vi "PIL_Main.vi"() -> ()   [LabVIEW 2018]
uses:
  controls/EXPERIMENT_Inputs.ctl
  controls/LASER_Inputs.ctl
  controls/LAMP_Inputs.ctl
  controls/GAS_Inputs.ctl
  controls/EXPERT_Inputs.ctl
  controls/DIGIT_5122_Inputs.ctl
  <instrlib>/niScope/Controls/niScope trigger source.ctl
  controls/HSDIO_6541_Inputs.ctl
  <instrlib>/niHSDIO/niHSDIO.llb/niHSDIO_ctl Trigger Source Values (Ring).ctl
  controls/SOFTWARE_Inputs.ctl
  controls/AO_6711_Inputs.ctl
  controls/AWG_5421_Inputs.ctl
  <instrlib>/niFgen/niFgen.llb/niFgen_ctl Trigger Source Values (Ring).ctl
  controls/XML_Inputs.ctl
  controls/VOLTAGES_Inputs.ctl
  controls/HEXA_Inputs.ctl
  controls/QUAD_Inputs.ctl
  controls/SEQUENCE_Inputs.ctl
  controls/EXCIT_Inputs.ctl
  controls/DATA_Inputs.ctl
  controls/TIMING_Inputs.ctl
  controls/PROCESSING_Inputs.ctl
  controls/TRAPPING_Inputs.ctl
  controls/SPECTRUM.ctl
  controls/EXCIT_Table.ctl
  controls/TIMING_Table.ctl
  controls/TIMING_Mandatory_Items.ctl
  controls/TIMING_Optional_Items.ctl
  controls/PIL_Status.ctl
  controls/QMH_UI_Cluster.ctl
  controls/QMH_UI_References.ctl
  controls/QMH_UI_Report.ctl
  controls/QMH_UI_Command.ctl
  controls/QMH_ICR_Command.ctl
  controls/QMH_Status.ctl
  controls/EXPERT_Path_Selector.ctl
  <vilib>/Utility/error.llb/DialogType.ctl
  Global_Variables.vi
panel:
  in  "Save As":bool
  in  "error in (no error)":errorcluster
  in  "Start":bool
  in  "Load":bool
  in  "Exit":bool
  in  "Tabs":T1(tab)
  out "SPECTRUM":T2={"Day Path"=path "D:/PIRENEA/DATA/2016/data_2016_01_01", "Spectrum Name"="2016_01_01_000.A00", "Accumulated"=FALSE, "Stored in Database"=FALSE, "From a Set of"=0, "Quality Flag"="Optimal"}
  in  "Change Experiment":bool
  out "EXPERIMENT Inputs":T3={"Setup"="", "Date"="", "User Name"="", "Comment"="", "Experiment Procedures"=[], "Chemical Source"="", "Sample Components"=[], "Species"=[], "Laser 1"={"Used"=TRUE, "Name"="Spectroscopy", "Wavelength"=1000.0, "Energy"=25.0}, "Laser 2"={"Used"=TRUE, "Name"="Spectroscopy", "Wavelength"=1000.0, "Energy"=25.0}, "Laser 3"={"Used"=TRUE, "Name"="Spectroscopy", "Wavelength"=1000.0, "Energy"=25.0}, "Laser 4"={"Used"=TRUE, "Name"="Spectroscopy", "Wavelength"=1000.0, "Energy"=25.0}, "Laser 5"={"Used"=TRUE, "Name"="Spectroscopy", "Wavelength"=1000.0, "Energy"=25.0}, "Lamp 1"={"Used"=TRUE, "Name"="Spectroscopy", "Wavelength"=1000.0, "Attenuation"=25.0}, "Lamp 2"={"Used"=TRUE, "Name"="Spectroscopy", "Wavelength"=1000.0, "Attenuation"=25.0}, "Gas 1"={"Used"=TRUE, "Name"="Spectroscopy", "Pressure"=1000.0}, "Gas 2"={"Used"=TRUE, "Name"="Spectroscopy", "Pressure"=1000.0}, "Gas 3"={"Used"=TRUE, "Name"="Spectroscopy", "Pressure"=1000.0}, "Gas 4"={"Used"=TRUE, "Name"="Spectroscopy", "Pressure"=1000.0}, "Gas 5"={"Used"=TRUE, "Name"="Spectroscopy", "Pressure"=1000.0}} caption="EXCIT Paths"
  in  "Change Voltages":bool
  out "VOLTAGES Inputs":T7={"Hexa 1"={"Used"=FALSE, "Voltage"=0.0}, "Hexa 2"={"Used"=FALSE, "Voltage"=0.0}, "Hexa 3"={"Used"=FALSE, "Voltage"=0.0}, "Quad 1"={"Used"=TRUE, "Voltage"=25.0}, "Quad 2"={"Used"=TRUE, "Voltage"=25.0}, "Quad 3"={"Used"=TRUE, "Voltage"=25.0}}
  out "SEQUENCE Inputs":T10={"EXCIT Inputs"={"Number of Excitations"=1, "Script Text"="script  excit1wfm\r    wait until scriptTrigger0\r    generate Sinus250to500a25dur1200fs10\rend script", "Table of Waveforms"=["Sinus250to500a25dur1200fs10"]}, "DATA Inputs"={"Record Length"=524000, "Sample Rate"=2000000.0, "Data Type"=0, "Vertical Range"=2.0, "Acquisition Duration"=100000.0}, "TIMING Inputs"={"Number of Acquisitions "=1, "Number of Accumulations"=1, "Table of Waveforms"=["", "", "", "", "", "", "", "", "", "", "", ""], "Script Text"=""}, "PROCESSING Inputs"={"Reference Mass"=300.0939, "Cyclotron Freq"=255.727, "Magnetron Freq"=0.001}, "TRAPPING Inputs"={"Number of Channels"=4, "Init Values"=[2.0, 9.0, 9.0, 2.0], "Opening Values"=[0.0, 0.0, 0.0, 0.0], "Trapping Values"=[2.0, 9.0, 9.0, 2.0], "Emptying Values"=[-10.0, -10.0, -10.0, -10.0], "Adiabatic ON"=FALSE, "Adiabatic Duration"=0, "Adiabatic Waveforms"=["Adiabatic_None_2_2_2000", "Adiabatic_Ramp_9_0_2000", "Adiabatic_DoubleRamp_9_0_2000", "Adiabatic_RC_2_0_2000.bin"], "Ions Refill ON"=FALSE, "Number of Ions Refills"=4, "Trapping Delay"=400.0, "Trapping Duration"=300.0}} {"TRAPPING Inputs"."Trapping Duration" min=2.0; "TRAPPING Inputs"."Trapping Delay" min=2.0; "TRAPPING Inputs"."Number of Ions Refills" min=1 max=1000; "TRAPPING Inputs"."Trapping Values" min=-10.0 max=10.0; "TRAPPING Inputs"."Init Values" min=-10.0 max=10.0; "TRAPPING Inputs"."Emptying Values" min=-10.0 max=10.0; "TRAPPING Inputs"."Opening Values" min=-10.0 max=10.0; "PROCESSING Inputs"."Magnetron Freq" format="%.5g"; "PROCESSING Inputs"."Cyclotron Freq" format="%.5g"; "PROCESSING Inputs"."Reference Mass" format="%.5g"; "TIMING Inputs"."Number of Accumulations" min=0 max=50 step=1; "TIMING Inputs"."Number of Acquisitions" min=1 max=10 step=1; "DATA Inputs"."Vertical Range" items=["0.2"=0.2, "0.4"=0.4, "1"=1.0, "2"=2.0, "4"=4.0, "10"=10.0]; "DATA Inputs"."Data Type" items=["I16", "DBL"]; "DATA Inputs"."Sample Rate" items=["1 MHz"=1000000.0, "2 MHz"=2000000.0, "5 MHz"=5000000.0, "10 MHz"=10000000.0, "20 MHz"=20000000.0, "25 MHz"=25000000.0, "50 MHz"=50000000.0, "100 MHz"=100000000.0]; "EXCIT Inputs"."Number of Excitations" min=1 max=10}
  in  "Change Sequence":bool
  in  "Change Expert":bool
  out "EXPERT Inputs":T16={"DIGIT 5122 Inputs"={"Sample Rate"=5000000.0, "Resource Name"="DIGIT_5122", "Channel Name"="0", "Trigger Source"="VAL_EXTERNAL", "Vertical Range"=2.0, "Trigger Level"=3.0}, "HSDIO 6541 Inputs"={"Resource Name"="HSDIO_6541", "Clock Rate"=1000000.0, "Trigger Source"="PFI0"}, "SOFTWARE Inputs"={"Application Directory"=path "D:/S.O.F.T.S/LABVIEW/PIL", "Software Version"="17.0f2", "Data Path"=path "D:/PIRENEA/DATA", "XML Path"=path "D:/PIRENEA/DATA", "XML File Filter"="*.xml", "XML Saved Path"=path "D:/PIRENEA/SAVED_XML", "Excit Scripts Path"=path "D:/PIRENEA/TECHNICAL/EXCIT_SCRIPTS", "Excit Scripts File Filter"="*.txt", "Excit Waveforms Path"=path "D:/PIRENEA/TECHNICAL/EXCIT_WFMS", "Excit Waveforms File Filter"="*.bin", "Timing Scripts Path"=path "D:/PIRENEA/TECHNICAL/TIMING_SCRIPTS", "Timing Scripts File Filter"="*.txt", "Timing Waveforms Path"=path "D:/PIRENEA/TECHNICAL/TIMING_WFMS", "Timing Waveforms File Filter"="*.bin", "Trapping Waveforms Path"=path "D:/PIRENEA/TECHNICAL/TRAPPING_WFMS", "Trapping Waveforms File Filter"="*.bin"}, "AO 6711 Inputs"={"Physical Channels"="AO_6711/ao0:3", "Min Voltage"=-10.0, "Max Voltage"=10.0, "Trigger Source"="/AO_6711/PFI3", "Counter"="AO_6711/ctr0"}, "AWG 5421 Inputs"={"Resource Name"="AWG_5421", "Sample Rate"=10000000.0, "Trigger Type"=2, "Trigger Source"="PFI0", "Waveform Gain"=0.31, "Digital Filter ON"=TRUE}, "XML Inputs"={"Version Tag Name"="XML_Version", "Version String"="1.1"}} {"AWG 5421 Inputs"."Sample Rate" format="%.2p"; "AWG 5421 Inputs"."Trigger Type" items=["None", "Software Edge", "Digital Edge", "Digital Level"]; "AO 6711 Inputs"."Max Voltage" min=-10.0 max=10.0; "AO 6711 Inputs"."Min Voltage" min=-10.0 max=10.0; "HSDIO 6541 Inputs"."Clock Rate" format="%.2p"; "DIGIT 5122 Inputs"."Trigger Level" format="%.2f"; "DIGIT 5122 Inputs"."Vertical Range" format="%.2f"; "DIGIT 5122 Inputs"."Sample Rate" step=65535.0 format="%#_3p"}
  in  "Excit Test":bool caption="AWG5421 Board"
  out "TIMING Script":string
  in  "Change Scientist":bool
  out "TIMING Table":T26={"Mandatory Items"={"Script Name"="", "GINI Time Period"=100.0, "HSDIO Delay"=60.0, "Shutter Duration before"=50.0, "Shutter Duration after"=50.0, "Filter Tau"=2.0, "Emtyping Duration"=1000.0}, "Optional Items"={"Eject"=0, "Acq"=0, "Excit"=0, "Gas"=0, "Laser"=0, "Lamp"=0}, "Times Table"=[["Excit1", "name", "Swift", "0.5", "1200", "70", "150", "550", "0", "0", "0"]]} {"Optional Items"."Laser" min=0 max=3; "Optional Items"."Gas" min=0 max=5; "Mandatory Items"."GINI Time Period" min=100000.0 max=1000000.0 format="%#_7g"; "Mandatory Items"."Shutter Duration after" min=2.0 max=100000.0; "Mandatory Items"."HSDIO Delay" min=0.0 max=100.0; "Mandatory Items"."Shutter Duration before" min=2.0 max=100000.0; "Mandatory Items"."Filter Tau" min=1000.0 max=2000.0; "Mandatory Items"."Emtyping Duration" min=2.0 format="%#_8g"}
  out "EXCIT Table":T29={"Number of Excits"=0, "Number of Ejects"=0, "Sampling Frequency"=0.0, "Waveforms Table"=[["Excit1", "name", "Swift", "0.5", "1200", "70", "150", "550", "0", "0", "0"]]}
  out "PIL Status":T30
  # "Lasers"
  # "nm"
  # "mJ"
  # "Lamps"
  # "nm"
  # "dB"
  # "Gas"
  # "bar"
  # "HEXAPOLE"
  # "QUADRIPOLE"
  # "GO_out"
  # "Gout"
  # "GI_in"
  # "Gin"
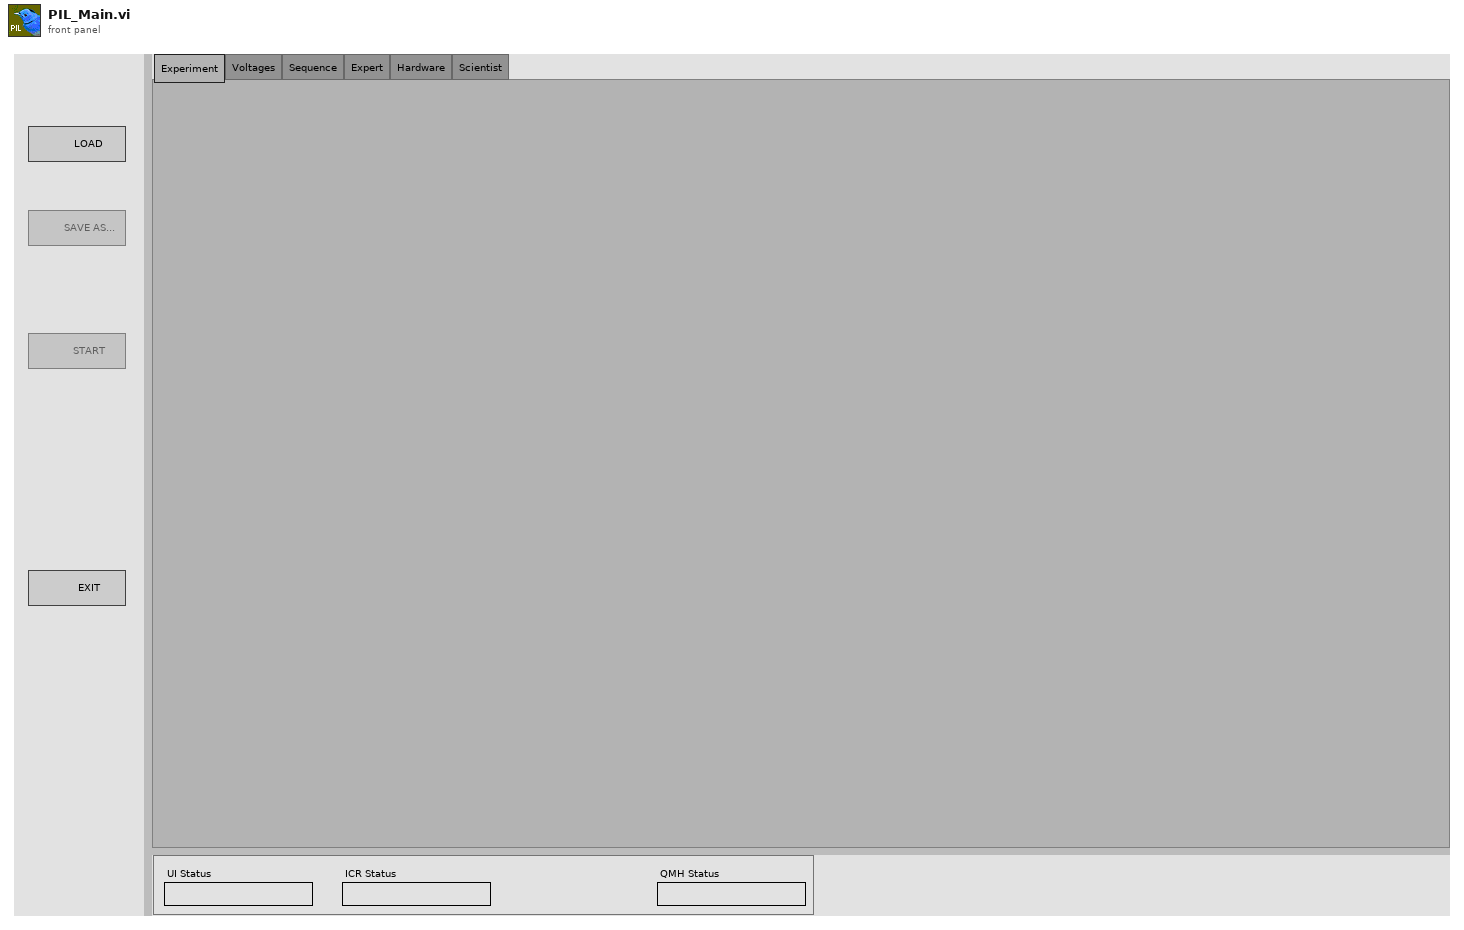
[diagram p1: front panel]
types:
  T1 = enum32{"Experiment", "Voltages", "Sequence", "Expert", "Hardware", "Scientist"}
  T2 = typedef "SPECTRUM.ctl" = cluster{"Day Path":path, "Spectrum Name":string, "Accumulated":bool, "Stored in Database":bool, "From a Set of":i16, "Quality Flag":string}
  T3 = typedef "EXPERIMENT_Inputs.ctl" = cluster{"Setup":string, "Date":string, "User Name":string, "Comment":string, "Experiment Procedures":string[], "Chemical Source":string, "Sample Components":string[], "Species":string[], "Laser 1":T4, "Laser 2":T4, "Laser 3":T4, "Laser 4":T4, "Laser 5":T4, "Lamp 1":T5, "Lamp 2":T5, "Gas 1":T6, "Gas 2":T6, "Gas 3":T6, "Gas 4":T6, "Gas 5":T6}
  T4 = typedef "LASER_Inputs.ctl" = cluster{"Used":bool, "Name":string, "Wavelength":dbl, "Energy":dbl}
  T5 = typedef "LAMP_Inputs.ctl" = cluster{"Used":bool, "Name":string, "Wavelength":dbl, "Attenuation":dbl}
  T6 = typedef "GAS_Inputs.ctl" = cluster{"Used":bool, "Name":string, "Pressure":dbl}
  T7 = typedef "VOLTAGES_Inputs.ctl" = cluster{"Hexa 1":T8, "Hexa 2":T8, "Hexa 3":T8, "Quad 1":T9, "Quad 2":T9, "Quad 3":T9}
  T8 = typedef "HEXA_Inputs.ctl" = cluster{"Used":bool, "Voltage":dbl}
  T9 = typedef "QUAD_Inputs.ctl" = cluster{"Used":bool, "Voltage":dbl}
  T10 = typedef "SEQUENCE_Inputs.ctl" = cluster{"EXCIT Inputs":T11, "DATA Inputs":T12, "TIMING Inputs":T13, "PROCESSING Inputs":T14, "TRAPPING Inputs":T15}
  T11 = typedef "EXCIT_Inputs.ctl" = cluster{"Number of Excitations":i32, "Script Text":string, "Table of Waveforms":string[]}
  T12 = typedef "DATA_Inputs.ctl" = cluster{"Record Length":i32, "Sample Rate":dbl, "Data Type":u8, "Vertical Range":dbl, "Acquisition Duration":dbl}
  T13 = typedef "TIMING_Inputs.ctl" = cluster{"Number of Acquisitions ":i16, "Number of Accumulations":i16, "Table of Waveforms":string[], "Script Text":string}
  T14 = typedef "PROCESSING_Inputs.ctl" = cluster{"Reference Mass":dbl, "Cyclotron Freq":dbl, "Magnetron Freq":dbl}
  T15 = typedef "TRAPPING_Inputs.ctl" = cluster{"Number of Channels":i32, "Init Values":dbl[], "Opening Values":dbl[], "Trapping Values":dbl[], "Emptying Values":dbl[], "Adiabatic ON":bool, "Adiabatic Duration":i32, "Adiabatic Waveforms":string[], "Ions Refill ON":bool, "Number of Ions Refills":i32, "Trapping Delay":dbl, "Trapping Duration":dbl}
  T16 = typedef "EXPERT_Inputs.ctl" = cluster{"DIGIT 5122 Inputs":T17, "HSDIO 6541 Inputs":T19, "SOFTWARE Inputs":T21, "AO 6711 Inputs":T22, "AWG 5421 Inputs":T23, "XML Inputs":T25}
  T17 = typedef "DIGIT_5122_Inputs.ctl" = cluster{"Sample Rate":dbl, "Resource Name":refnum<k15>, "Channel Name":string, "Trigger Source":T18, "Vertical Range":dbl, "Trigger Level":dbl}
  T18 = typedef "niScope trigger source.ctl" = string
  T19 = typedef "HSDIO_6541_Inputs.ctl" = cluster{"Resource Name":refnum<k15>, "Clock Rate":dbl, "Trigger Source":T20}
  T20 = typedef "niHSDIO_ctl Trigger Source Values (Ring).ctl" = string
  T21 = typedef "SOFTWARE_Inputs.ctl" = cluster{"Application Directory":path, "Software Version":string, "Data Path":path, "XML Path":path, "XML File Filter":string, "XML Saved Path":path, "Excit Scripts Path":path, "Excit Scripts File Filter":string, "Excit Waveforms Path":path, "Excit Waveforms File Filter":string, "Timing Scripts Path":path, "Timing Scripts File Filter":string, "Timing Waveforms Path":path, "Timing Waveforms File Filter":string, "Trapping Waveforms Path":path, "Trapping Waveforms File Filter":string}
  T22 = typedef "AO_6711_Inputs.ctl" = cluster{"Physical Channels":tag, "Min Voltage":dbl, "Max Voltage":dbl, "Trigger Source":tag, "Counter":tag}
  T23 = typedef "AWG_5421_Inputs.ctl" = cluster{"Resource Name":refnum<k15>, "Sample Rate":dbl, "Trigger Type":u16, "Trigger Source":T24, "Waveform Gain":dbl, "Digital Filter ON":bool}
  T24 = typedef "niFgen_ctl Trigger Source Values (Ring).ctl" = string
  T25 = typedef "XML_Inputs.ctl" = cluster{"Version Tag Name":string, "Version String":string}
  T26 = typedef "TIMING_Table.ctl" = cluster{"Mandatory Items":T27, "Optional Items":T28, "Times Table":string[][]}
  T27 = typedef "TIMING_Mandatory_Items.ctl" = cluster{"Script Name":string, "GINI Time Period":dbl, "HSDIO Delay":dbl, "Shutter Duration before":dbl, "Shutter Duration after":dbl, "Filter Tau":dbl, "Emtyping Duration":dbl}
  T28 = typedef "TIMING_Optional_Items.ctl" = cluster{"Eject":u32, "Acq":i32, "Excit":u32, "Gas":i32, "Laser":i32, "Lamp":i32}
  T29 = typedef "EXCIT_Table.ctl" = cluster{"Number of Excits":u16, "Number of Ejects":u16, "Sampling Frequency":dbl, "Waveforms Table":string[][]}
  T30 = typedef "PIL_Status.ctl" = cluster{"UI Status":string, "ICR Status":string, "QMH Status":string}
  T31 = typedef "QMH_UI_Cluster.ctl" = cluster{"QMH UI References":T32, "QMH UI Report":T33}
  T32 = typedef "QMH_UI_References.ctl" = cluster{"Refnum Load":refnum<vi>, "Refnum Save As":refnum<vi>, "Refnum Start":refnum<vi>, "Refnum Exit":refnum<vi>, "Refnum Tabs":refnum<vi>, "Refnum SPECTRUM":refnum<vi>, "Refnum EXPERIMENT":refnum<vi>, "Refnum VOLTAGES":refnum<vi>, "Refnum SEQUENCE":refnum<vi>, "Refnum EXPERT":refnum<vi>, "Refnum EXCIT Table":refnum<vi>, "Refnum TIMING Table":refnum<vi>, "Refnum CHANGE Experiment":refnum<vi>, "Refnum CHANGE Voltages":refnum<vi>, "Refnum CHANGE Sequence":refnum<vi>, "Refnum CHANGE Expert":refnum<vi>, "Refnum CHANGE Scientist":refnum<vi>, "Refnum PIL Status":refnum<vi>}
  T33 = typedef "QMH_UI_Report.ctl" = cluster{"UI Status":T34, "ICR Status":T35, "QMH Status":T36}
  T34 = typedef "QMH_UI_Command.ctl" = enum16{"Initialize", "UI Load", "UI Save", "UI Save As", "UI Change Experiment", "UI Change Voltages", "UI Change Sequence", "UI Change Expert", "UI Change Scientist", "Ready to Start", "UI Start", "Waiting for ICR", "UI Exit", "Update Report", "Update ICR Status", "Waiting for User"}
  T35 = typedef "QMH_ICR_Command.ctl" = enum16{"Initialize", "Sequence Setup", "ICR Start", "ICR Stop", "Hardware Setup", "Next Accumulation", "Waiting for Trigger", "Sequence Started", "Sequence Finished", "Writing Data", "Hardware Reset", "Exit"}
  T36 = typedef "QMH_Status.ctl" = enum16{"Init", "Loading", "Setup", "Ready to Start", "Started", "Idle"}
  T37 = typedef "EXPERT_Path_Selector.ctl" = enum16{"Application", "Resources", "Data", "XML", "XML Saved", "Load Directory"}
  T38 = typedef "QMH_UI_Message.ctl" = cluster{"Command":T34, "Data":variant}
  T39 = typedef "DialogType.ctl" = u16
  T40 = enum32{"invalid app kind", "Development System", "Run Time System", "Student Edition", "Embedded LabVIEW", "Evaluation", "Custom"}
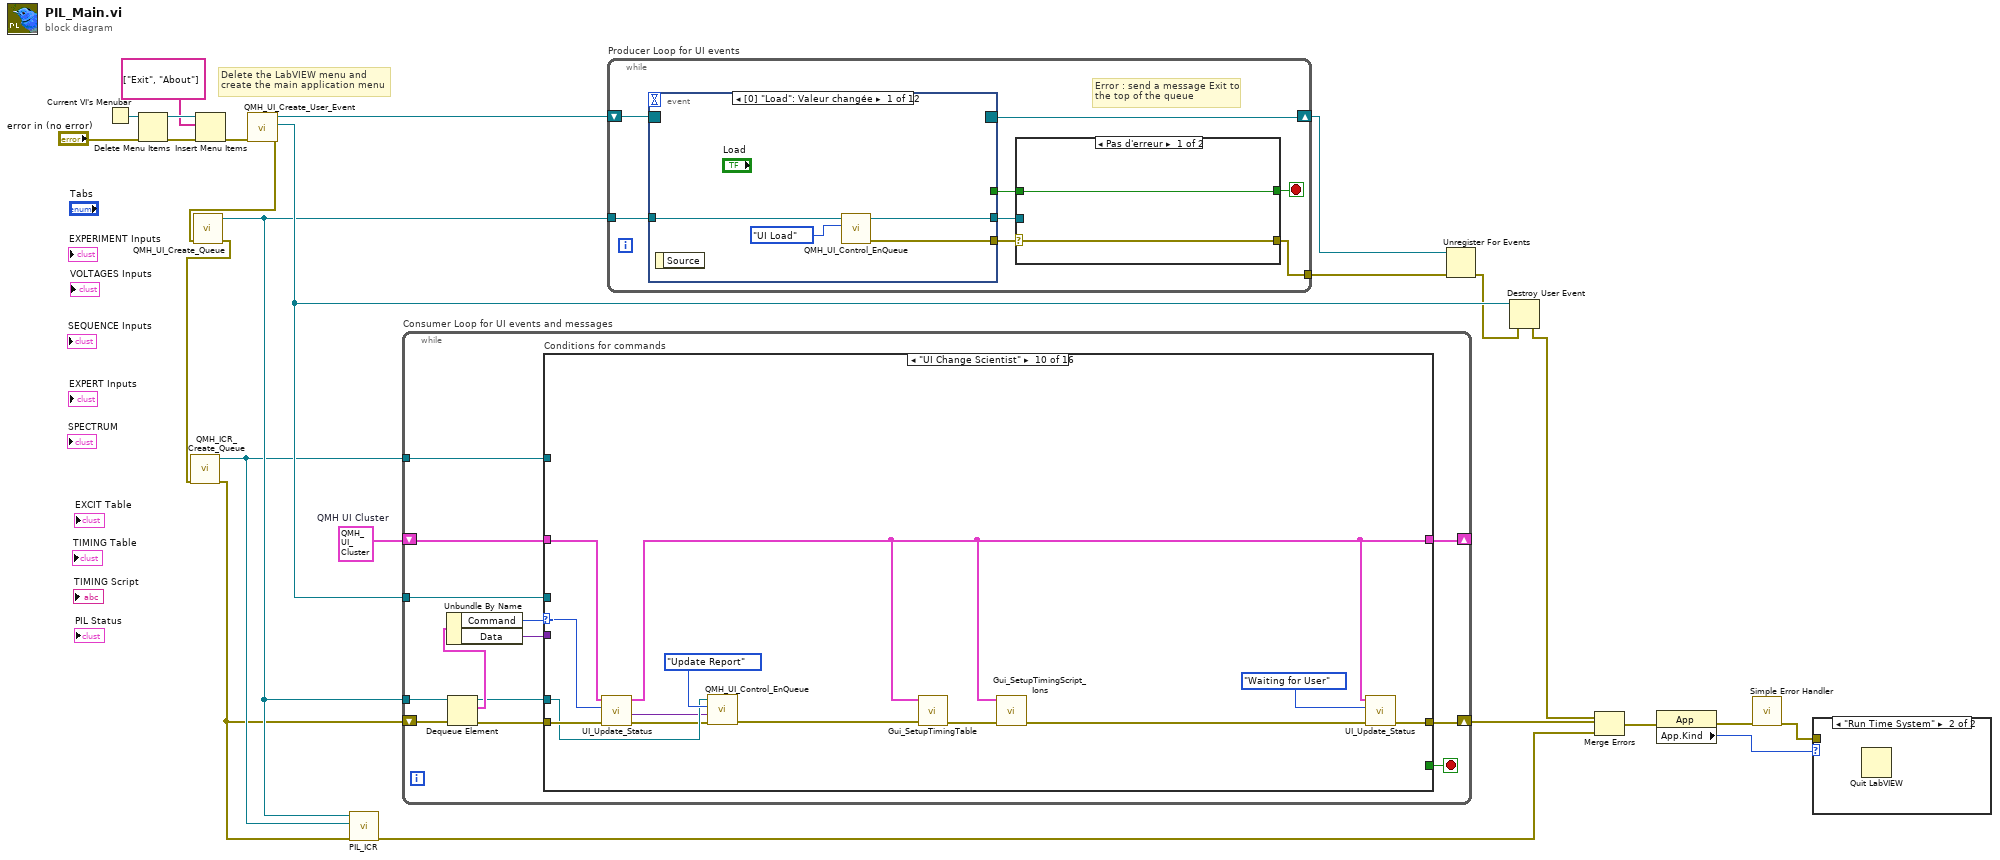
[diagram p0: block diagram]
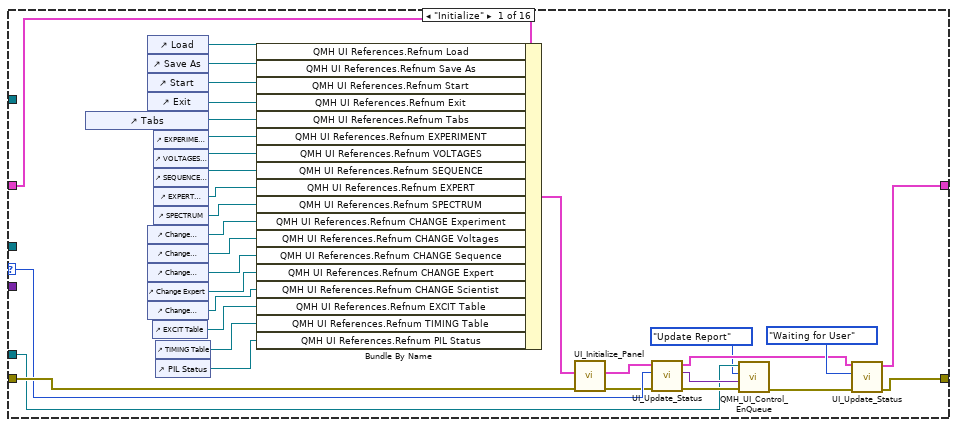
[diagram p2: hidden frame]
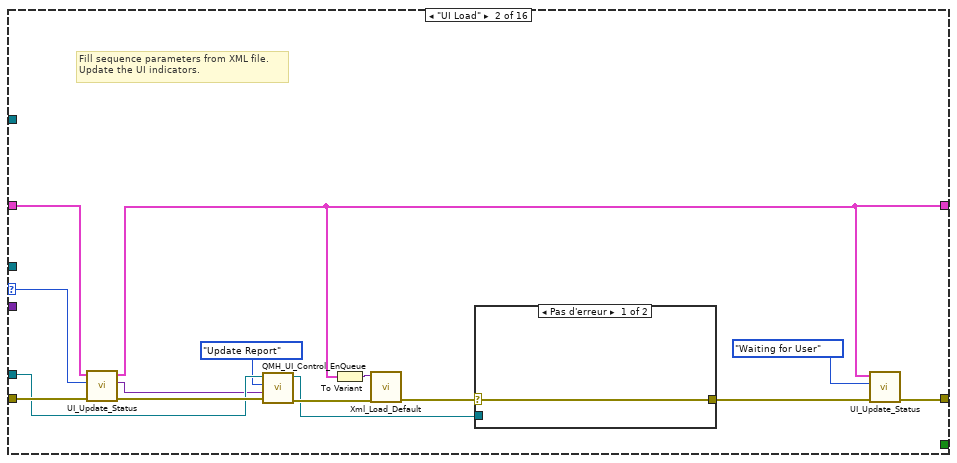
[diagram p3: hidden frame]
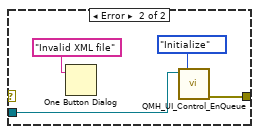
[diagram p4: hidden frame]
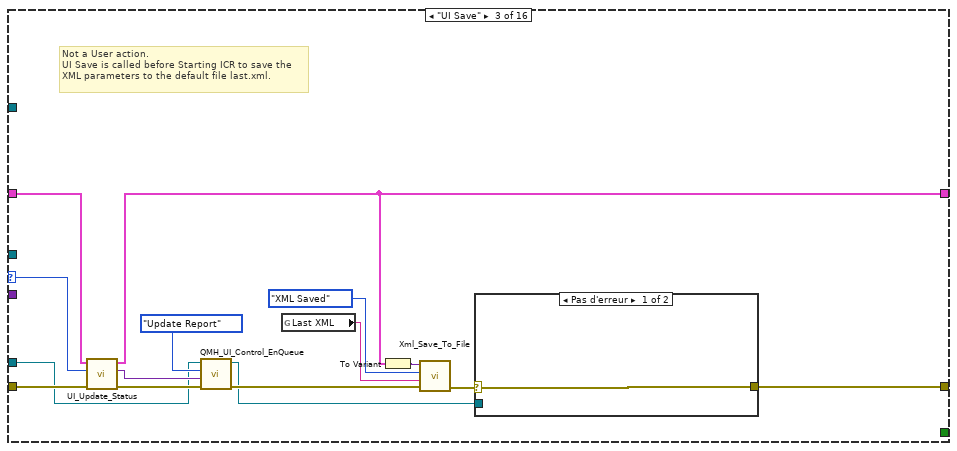
[diagram p5: hidden frame]
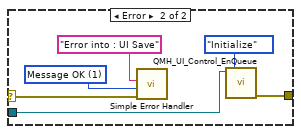
[diagram p6: hidden frame]
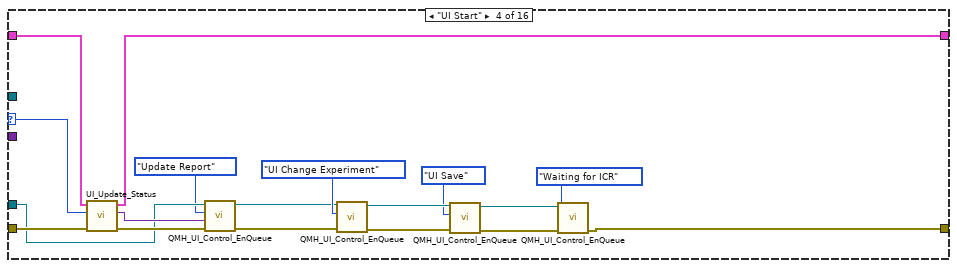
[diagram p7: hidden frame]
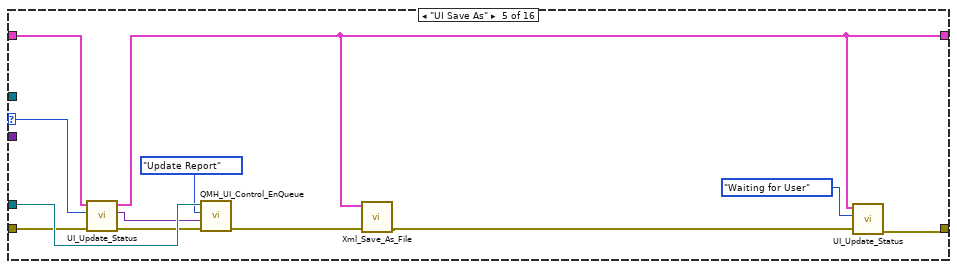
[diagram p8: hidden frame]
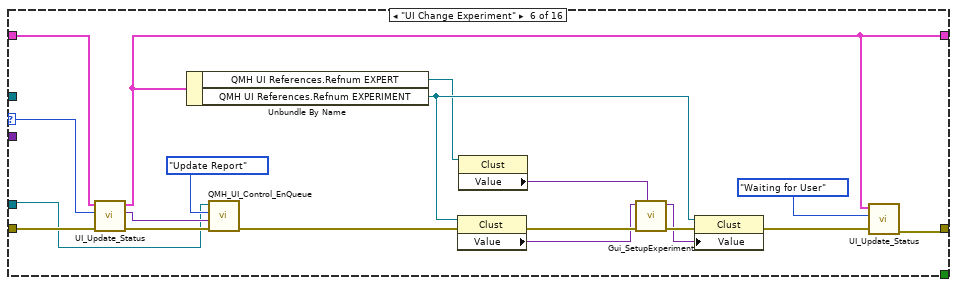
[diagram p9: hidden frame]
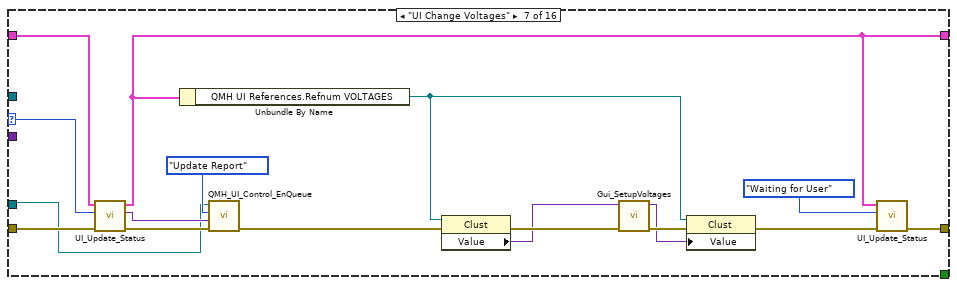
[diagram p10: hidden frame]
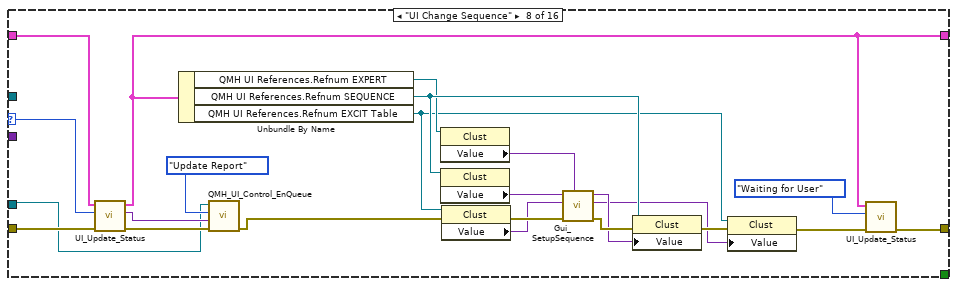
[diagram p11: hidden frame]
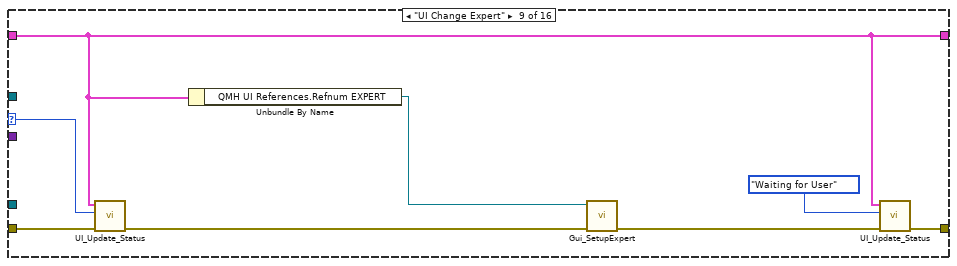
[diagram p12: hidden frame]
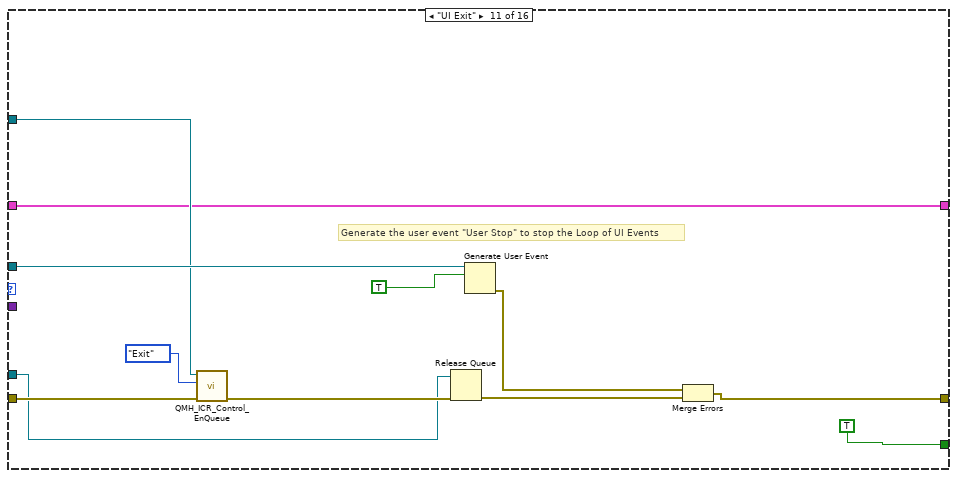
[diagram p13: hidden frame]
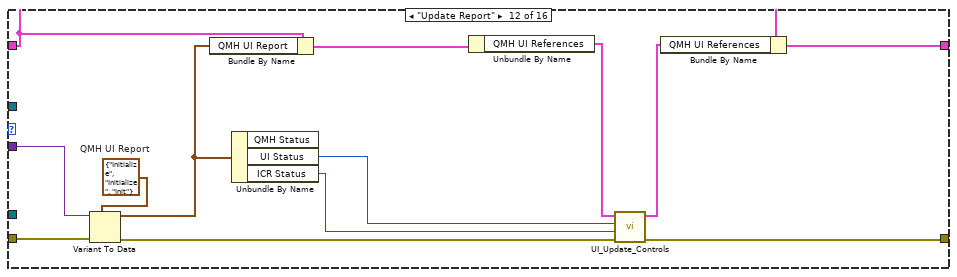
[diagram p14: hidden frame]
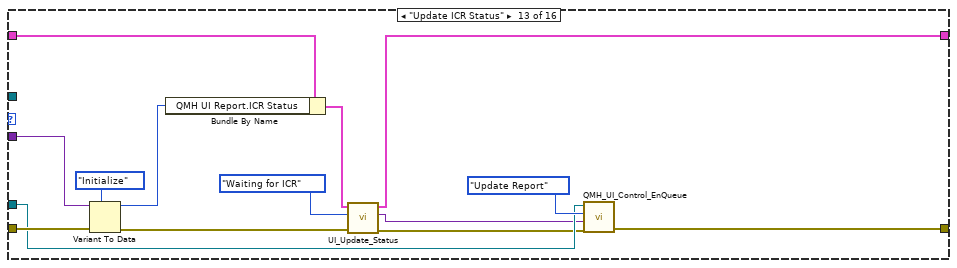
[diagram p15: hidden frame]
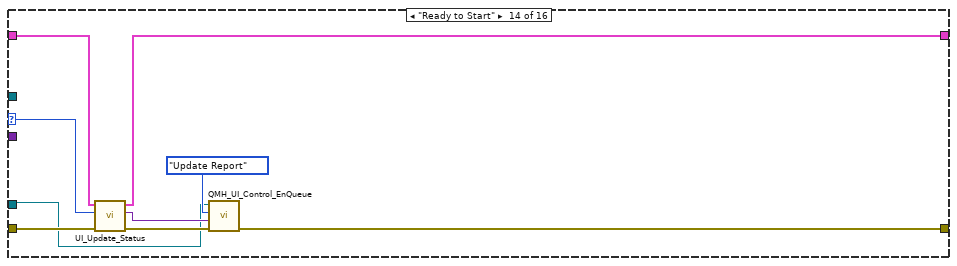
[diagram p16: hidden frame]
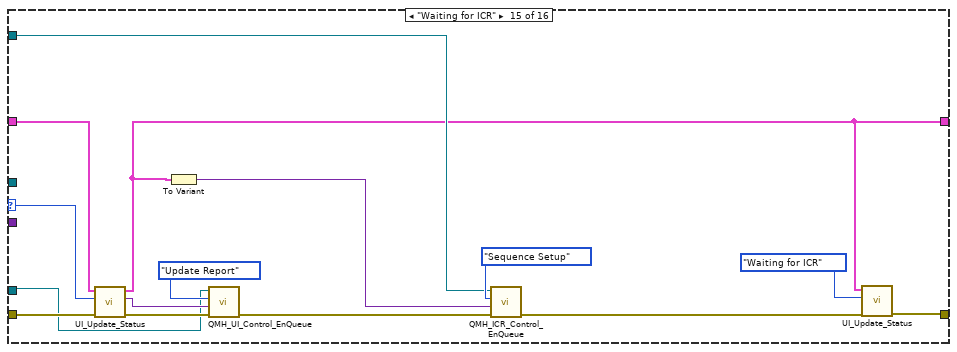
[diagram p17: hidden frame]
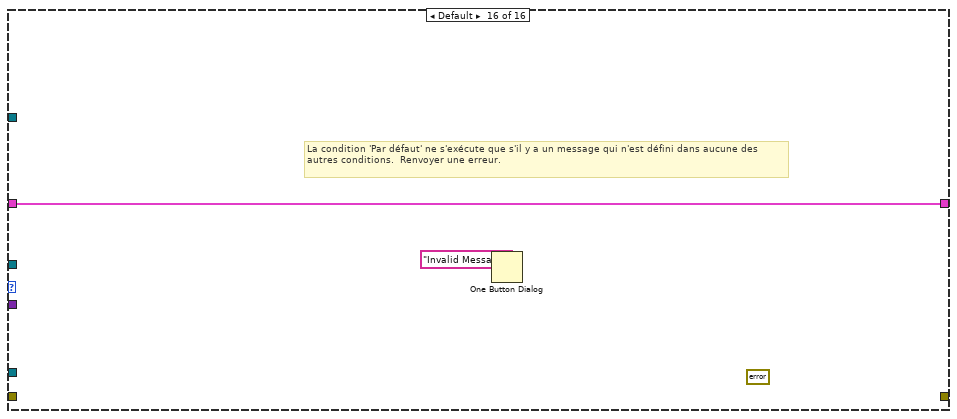
[diagram p18: hidden frame]
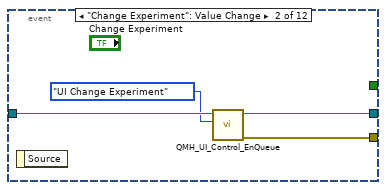
[diagram p19: hidden frame]
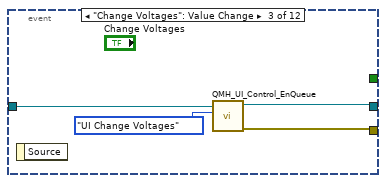
[diagram p20: hidden frame]
diagram:
  w23 = T31 {"QMH UI References"={"Refnum Load"=refnum, "Refnum Save As"=refnum, "Refnum Start"=refnum, "Refnum Exit"=refnum, "Refnum Tabs"=refnum, "Refnum SPECTRUM"=refnum, "Refnum EXPERIMENT"=refnum, "Refnum VOLTAGES"=refnum, "Refnum SEQUENCE"=refnum, "Refnum EXPERT"=refnum, "Refnum EXCIT Table"=refnum, "Refnum TIMING Table"=refnum, "Refnum CHANGE Experiment"=refnum, "Refnum CHANGE Voltages"=refnum, "Refnum CHANGE Sequence"=refnum, "Refnum CHANGE Expert"=refnum, "Refnum CHANGE Scientist"=refnum, "Refnum PIL Status"=refnum}, "QMH UI Report"={"UI Status"=enum."Initialize", "ICR Status"=enum."Initialize", "QMH Status"=enum."Init"}}  # QMH UI Cluster
  # "Delete the LabVIEW menu and\ncreate the main application menu"
  n1 = Current VI's Menubar() -> (w6:refnum<k9>)
  n2 = Delete Menu Items(6:"error in (no error)", 9:w6) -> (0:w5:errorcluster, 3:w4:refnum<k9>)  [unwired: 2 in]
  n3 = Insert Menu Items(6:w5, 8:string[] ["Exit", "About"] ("noms des éléments"), 9:w4) -> (0:w2:errorcluster)  [unwired: 3 in, 2 out]
  n4 = call "QMH_UI_Create_User_Event.vi"("error in (no error)"=w2) -> ("error out"=w22:errorcluster, "User Stop Event"=w18:refnum<user-event>, "Refnum register for events"=w24:refnum<event-registration>)  [unwired: 8 in]
  n5 = call "QMH_UI_Create_Queue.vi"("error in (no error)"=w22) -> ("error out"=w8:errorcluster, "UI Queue"=w11:refnum<queue>)  [unwired: 9 in]
  n6 = call "QMH_ICR_Create_Queue.vi"("error in (no error)"=w8) -> ("error out"=w7:errorcluster, "ICR Queue"=w10:refnum<queue>)  [unwired: 9 in]
  n7 = call "PIL_ICR.vi"("error in (no error)"=w7, "ICR Queue"=w10, "UI Queue"=w11) -> ("error out"=w9:errorcluster)  [unwired: 8 in]
  n8 = while "Consumer Loop for UI events and messages" {
    shift-right: [w28] -> _
    shift-left: w23 -> [w37]
    shift-right: [w26] -> w19
    shift-left: w7 -> [w33]
    tunnel: w11 -> [w34]
    tunnel: w18 -> [w29]
    tunnel: w10 -> [w25]
    stop <- w36 stop-if-true
    n9 = Dequeue Element(queue=w34, error in (no error)=w33) -> (queue out=w32:refnum<queue>, element=w35:T38, error out=w27:errorcluster)  [unwired: 2 out]
    n10 = Unbundle By Name(w35) -> ("Command"=w31:T34, "Data"=w30:variant)
    n11 = case "Conditions for commands" shown="\"UI Change Scientist\"" w31 {
      selector: w31 -> [w50 w84 w102 w129 w138 w156 w173 w196 w208 w220 _ _ _ w266 w281 _]
      tunnel: w32 -> [w39 w75 w95 w120 w142 w154 w171 w194 _ w215 w225 _ w254 w264 w279 _]
      tunnel: w37 -> [w68 w79 w101 w128 w137 w157 w174 w197 w202 w217 w223 w237 w259 w267 w282 w286]
      tunnel: [_ _ _ _ _ _ _ _ _ _ TRUE _ _ _ _ _] -> w36
      tunnel: w30 -> [_ _ _ _ _ _ _ _ _ _ _ w247 w261 _ _ _]
      tunnel: w29 -> [_ _ _ _ _ _ _ _ _ _ w231 _ _ _ _ _]
      tunnel: [w46 w72 w91 w115 w131 w143 w162 w180 w202 w210 w223 w243 w251 w263 w271 w286] -> w28
      tunnel: w27 -> [w51 w85 w103 w130 w139 w155 w172 w195 w207 w221 w227 w242 w260 w265 w280 _]
      tunnel: [w49 w80 w96 w113 w133 w144 w163 w181 w203 w219 w229 w241 w255 w262 w272 _] -> w26
      tunnel: w25 -> [_ _ _ _ _ _ _ _ _ _ w224 _ _ _ w277 _]
      frame "Initialize" {
        n12 = control-ref of="Tabs"() -> (w67:refnum<vi>)
        n13 = control-ref of="Load"() -> (w70:refnum<vi>)
        n14 = control-ref of="Save As"() -> (w57:refnum<vi>)
        n15 = control-ref of="Start"() -> (w58:refnum<vi>)
        n16 = control-ref of="Exit"() -> (w69:refnum<vi>)
        n17 = control-ref of="Change Experiment"() -> (w62:refnum<vi>)
        n18 = control-ref of="Change Voltages"() -> (w59:refnum<vi>)
        n19 = control-ref of="Change Sequence"() -> (w60:refnum<vi>)
        n20 = control-ref of="Change Expert"() -> (w61:refnum<vi>)
        n21 = control-ref of="Change Scientist"() -> (w54:refnum<vi>)
        n22 = control-ref of="EXCIT Table"() -> (w53:refnum<vi>)
        n23 = control-ref of="EXPERIMENT Inputs"() -> (w66:refnum<vi>)
        n24 = control-ref of="VOLTAGES Inputs"() -> (w65:refnum<vi>)
        n25 = control-ref of="SEQUENCE Inputs"() -> (w64:refnum<vi>)
        n26 = control-ref of="EXPERT Inputs"() -> (w56:refnum<vi>)
        n27 = control-ref of="SPECTRUM"() -> (w63:refnum<vi>)
        n28 = control-ref of="TIMING Table"() -> (w55:refnum<vi>)
        n29 = control-ref of="PIL Status"() -> (w52:refnum<vi>)
        n30 = Bundle By Name(cluster=w68, "QMH UI References.Refnum Load"=w70, "QMH UI References.Refnum Save As"=w57, "QMH UI References.Refnum Start"=w58, "QMH UI References.Refnum Exit"=w69, "QMH UI References.Refnum Tabs"=w67, "QMH UI References.Refnum EXPERIMENT"=w66, "QMH UI References.Refnum VOLTAGES"=w65, "QMH UI References.Refnum SEQUENCE"=w64, "QMH UI References.Refnum EXPERT"=w56, "QMH UI References.Refnum SPECTRUM"=w63, "QMH UI References.Refnum CHANGE Experiment"=w62, "QMH UI References.Refnum CHANGE Voltages"=w59, "QMH UI References.Refnum CHANGE Sequence"=w60, "QMH UI References.Refnum CHANGE Expert"=w61, "QMH UI References.Refnum CHANGE Scientist"=w54, "QMH UI References.Refnum EXCIT Table"=w53, "QMH UI References.Refnum TIMING Table"=w55, "QMH UI References.Refnum PIL Status"=w52) -> (w44:T31)
        n31 = call "UI_Initialize_Panel.vi"("error in (no error)"=w51, "QMH UI Cluster"=w44) -> ("error out"=w45:errorcluster, "QMH UI Cluster"=w43:T31)  [unwired: 8 in]
        n32 = call "UI_Update_Status.vi"("error in (no error)"=w45, "UI Status"=w50, "QMH UI Cluster"=w43) -> ("error out"=w42:errorcluster, "Variant"=w41:variant, "QMH UI Cluster"=w47:T31)  [unwired: 6 in]
        n33 = call "QMH_UI_Control_EnQueue.vi"("error in (no error)"=w42, "Variant"=w41, "Command"=QMH_UI_Command."Update Report", "UI Queue"=w39) -> ("error out"=w40:errorcluster)  [unwired: 6 in, 1 out]
        n34 = call "UI_Update_Status.vi"("error in (no error)"=w40, "UI Status"=QMH_UI_Command."Waiting for User", "QMH UI Cluster"=w47) -> ("error out"=w49:errorcluster, "QMH UI Cluster"=w46:T31)  [unwired: 6 in, 1 out]
      }
      frame "UI Load" {
        # "Fill sequence parameters from XML file.\nUpdate the UI indicators."
        n35 = call "UI_Update_Status.vi"("error in (no error)"=w85, "UI Status"=w84, "QMH UI Cluster"=w79) -> ("error out"=w77:errorcluster, "Variant"=w71:variant, "QMH UI Cluster"=w72:T31)  [unwired: 6 in]
        n36 = call "QMH_UI_Control_EnQueue.vi"("error in (no error)"=w77, "Variant"=w71, "Command"=QMH_UI_Command."Update Report", "UI Queue"=w75) -> ("error out"=w76:errorcluster, "UI Queue"=w74:refnum<queue>)  [unwired: 6 in]
        n37 = To Variant(anything=w72) -> (Variant=w83:variant)
        n38 = call "Xml_Load_Default.vi"("error in (no error)"=w76, "Variant"=w83) -> ("error out"=w81:errorcluster)  [unwired: 9 in]
        n39 = case shown="Pas d'erreur" w81 {
          selector: w81 -> [w86 _]
          tunnel: [w86 w90] -> w82
          tunnel: w74 -> [_ w87]
          frame No Error {
          }
          frame Error {
            n40 = One Button Dialog(message="Invalid XML file") -> ()  [unwired: 1 in, 1 out]
            n41 = call "QMH_UI_Control_EnQueue.vi"("Command"=QMH_UI_Command."Initialize", "UI Queue"=w87) -> ("error out"=w90:errorcluster)  [unwired: 8 in, 1 out]
          }
        }
        n42 = call "UI_Update_Status.vi"("error in (no error)"=w82, "UI Status"=QMH_UI_Command."Waiting for User", "QMH UI Cluster"=w72) -> ("error out"=w80:errorcluster)  [unwired: 6 in, 2 out]
      }
      frame "UI Save" {
        # "Not a User action.\nUI Save is called before Starting ICR to save the\nXML parameters to the default file last.xml."
        n43 = call "UI_Update_Status.vi"("error in (no error)"=w103, "UI Status"=w102, "QMH UI Cluster"=w101) -> ("error out"=w104:errorcluster, "Variant"=w100:variant, "QMH UI Cluster"=w91:T31)  [unwired: 6 in]
        n44 = call "QMH_UI_Control_EnQueue.vi"("error in (no error)"=w104, "Variant"=w100, "Command"=QMH_UI_Command."Update Report", "UI Queue"=w95) -> ("error out"=w99:errorcluster, "UI Queue"=w92:refnum<queue>)  [unwired: 6 in]
        n45 = global read "Global_Variables.vi" "Last XML"() -> (w93:string)
        n46 = To Variant(anything=w91) -> (Variant=w98:variant)
        n47 = call "Xml_Save_To_File.vi"("error in (no error)"=w99, "Filename"=w93, "EXPERT Path Selector"=EXPERT_Path_Selector."XML Saved", "Variant"=w98) -> ("error out"=w97:errorcluster)  [unwired: 7 in]
        n48 = case shown="Pas d'erreur" w97 {
          selector: w97 -> [w106 w109]
          tunnel: [w106 w112] -> w96
          tunnel: w92 -> [_ w110]
          frame No Error {
          }
          frame Error {
            w107 = T39 1 items=["pas de dialogue", "Message OK", "Message continuer ou arrêter", "Message OK + mises en garde", "Arrêter/Continuer + mises en garde"] ("type of dialog (OK msg:1)")
            n49 = call <vilib>:"Simple Error Handler.vi"("error source (\" \")"="Error into : UI Save" ("error source (\" \")"), "type of dialog (OK msg:1)"=w107, "error in (no error)"=w109) -> ()  [unwired: 2 in, 5 out]
            n50 = call "QMH_UI_Control_EnQueue.vi"("Command"=QMH_UI_Command."Initialize", "UI Queue"=w110) -> ("error out"=w112:errorcluster)  [unwired: 8 in, 1 out]
          }
        }
      }
      frame "UI Start" {
        n51 = call "UI_Update_Status.vi"("error in (no error)"=w130, "UI Status"=w129, "QMH UI Cluster"=w128) -> ("error out"=w123:errorcluster, "Variant"=w121:variant, "QMH UI Cluster"=w115:T31)  [unwired: 6 in]
        n52 = call "QMH_UI_Control_EnQueue.vi"("error in (no error)"=w123, "Variant"=w121, "Command"=QMH_UI_Command."Update Report", "UI Queue"=w120) -> ("error out"=w122:errorcluster, "UI Queue"=w119:refnum<queue>)  [unwired: 6 in]
        n53 = call "QMH_UI_Control_EnQueue.vi"("error in (no error)"=w122, "Command"=QMH_UI_Command."UI Change Experiment", "UI Queue"=w119) -> ("error out"=w126:errorcluster, "UI Queue"=w125:refnum<queue>)  [unwired: 7 in]
        n54 = call "QMH_UI_Control_EnQueue.vi"("error in (no error)"=w126, "Command"=QMH_UI_Command."UI Save", "UI Queue"=w125) -> ("error out"=w114:errorcluster, "UI Queue"=w117:refnum<queue>)  [unwired: 7 in]
        n55 = call "QMH_UI_Control_EnQueue.vi"("error in (no error)"=w114, "Command"=QMH_UI_Command."Waiting for ICR", "UI Queue"=w117) -> ("error out"=w113:errorcluster)  [unwired: 7 in, 1 out]
      }
      frame "UI Save As" {
        n56 = call "UI_Update_Status.vi"("error in (no error)"=w139, "UI Status"=w138, "QMH UI Cluster"=w137) -> ("error out"=w140:errorcluster, "Variant"=w136:variant, "QMH UI Cluster"=w131:T31)  [unwired: 6 in]
        n57 = call "QMH_UI_Control_EnQueue.vi"("error in (no error)"=w140, "Variant"=w136, "Command"=QMH_UI_Command."Update Report", "UI Queue"=w142) -> ("error out"=w135:errorcluster)  [unwired: 6 in, 1 out]
        n58 = call "Xml_Save_As_File.vi"("error in (no error)"=w135, "QMH UI Cluster"=w131) -> ("error out"=w134:errorcluster)  [unwired: 9 in]
        n59 = call "UI_Update_Status.vi"("error in (no error)"=w134, "UI Status"=QMH_UI_Command."Waiting for User", "QMH UI Cluster"=w131) -> ("error out"=w133:errorcluster)  [unwired: 6 in, 2 out]
      }
      frame "UI Change Experiment" {
        n60 = call "UI_Update_Status.vi"("error in (no error)"=w155, "UI Status"=w156, "QMH UI Cluster"=w157) -> ("error out"=w159:errorcluster, "Variant"=w158:variant, "QMH UI Cluster"=w143:T31)  [unwired: 6 in]
        n61 = Unbundle By Name(w143) -> ("QMH UI References.Refnum EXPERT"=w148:refnum<vi>, "QMH UI References.Refnum EXPERIMENT"=w153:refnum<vi>)
        n62 = call "QMH_UI_Control_EnQueue.vi"("error in (no error)"=w159, "Variant"=w158, "Command"=QMH_UI_Command."Update Report", "UI Queue"=w154) -> ("error out"=w152:errorcluster)  [unwired: 6 in, 1 out]
        n63 = property class="Clust"(reference=w153, error in=w152) -> (error out=w151:errorcluster, "Value"=w150:variant)  [unwired: 1 out]
        n64 = property class="Clust"(reference=w148) -> ("Value"=w147:variant)  [unwired: 1 in, 2 out]
        n65 = call "Gui_SetupExperiment.vi"("Variant for Path"=w147, "error in (no error)"=w151, "Variant"=w150) -> ("error out"=w161:errorcluster, "Variant Output"=w149:variant)  [unwired: 7 in]
        n66 = property class="Clust"(reference=w153, error in=w161, "Value"=w149) -> (error out=w145:errorcluster)  [unwired: 1 out]
        n67 = call "UI_Update_Status.vi"("error in (no error)"=w145, "UI Status"=QMH_UI_Command."Waiting for User", "QMH UI Cluster"=w143) -> ("error out"=w144:errorcluster)  [unwired: 6 in, 2 out]
      }
      frame "UI Change Voltages" {
        n68 = call "UI_Update_Status.vi"("error in (no error)"=w172, "UI Status"=w173, "QMH UI Cluster"=w174) -> ("error out"=w176:errorcluster, "Variant"=w175:variant, "QMH UI Cluster"=w162:T31)  [unwired: 6 in]
        n69 = Unbundle By Name(w162) -> ("QMH UI References.Refnum VOLTAGES"=w170:refnum<vi>)
        n70 = call "QMH_UI_Control_EnQueue.vi"("error in (no error)"=w176, "Variant"=w175, "Command"=QMH_UI_Command."Update Report", "UI Queue"=w171) -> ("error out"=w169:errorcluster)  [unwired: 6 in, 1 out]
        n71 = property class="Clust"(reference=w170, error in=w169) -> (error out=w168:errorcluster, "Value"=w167:variant)  [unwired: 1 out]
        n72 = call "Gui_SetupVoltages.vi"("error in (no error)"=w168, "Variant"=w167) -> ("error out"=w178:errorcluster, "Variant Output"=w166:variant)  [unwired: 8 in]
        n73 = property class="Clust"(reference=w170, error in=w178, "Value"=w166) -> (error out=w164:errorcluster)  [unwired: 1 out]
        n74 = call "UI_Update_Status.vi"("error in (no error)"=w164, "UI Status"=QMH_UI_Command."Waiting for User", "QMH UI Cluster"=w162) -> ("error out"=w163:errorcluster)  [unwired: 6 in, 2 out]
      }
      frame "UI Change Sequence" {
        n75 = call "UI_Update_Status.vi"("error in (no error)"=w195, "UI Status"=w196, "QMH UI Cluster"=w197) -> ("error out"=w199:errorcluster, "Variant"=w198:variant, "QMH UI Cluster"=w180:T31)  [unwired: 6 in]
        n76 = Unbundle By Name(w180) -> ("QMH UI References.Refnum EXPERT"=w190:refnum<vi>, "QMH UI References.Refnum SEQUENCE"=w193:refnum<vi>, "QMH UI References.Refnum EXCIT Table"=w183:refnum<vi>)
        n77 = call "QMH_UI_Control_EnQueue.vi"("error in (no error)"=w199, "Variant"=w198, "Command"=QMH_UI_Command."Update Report", "UI Queue"=w194) -> ("error out"=w188:errorcluster)  [unwired: 6 in, 1 out]
        n78 = property class="Clust"(reference=w190) -> ("Value"=w189:variant)  [unwired: 1 in, 2 out]
        n79 = property class="Clust"(reference=w193) -> ("Value"=w192:variant)  [unwired: 1 in, 2 out]
        n80 = property class="Clust"(reference=w183, error in=w188) -> (error out=w187:errorcluster, "Value"=w186:variant)  [unwired: 1 out]
        n81 = call "Gui_SetupSequence.vi"("Variant For Path"=w189, "error in (no error)"=w187, "Excit Table Variant"=w186, "Variant"=w192) -> ("error out"=w201:errorcluster, "Excit Table Variant Output"=w182:variant, "Variant Output"=w191:variant)  [unwired: 5 in]
        n82 = property class="Clust"(reference=w193, error in=w201, "Value"=w191) -> (error out=w185:errorcluster)  [unwired: 1 out]
        n83 = property class="Clust"(reference=w183, error in=w185, "Value"=w182) -> (error out=w184:errorcluster)  [unwired: 1 out]
        n84 = call "UI_Update_Status.vi"("error in (no error)"=w184, "UI Status"=QMH_UI_Command."Waiting for User", "QMH UI Cluster"=w180) -> ("error out"=w181:errorcluster)  [unwired: 6 in, 2 out]
      }
      frame "UI Change Expert" {
        n85 = call "UI_Update_Status.vi"("error in (no error)"=w207, "UI Status"=w208, "QMH UI Cluster"=w202) -> ("error out"=w209:errorcluster)  [unwired: 6 in, 2 out]
        n86 = Unbundle By Name(w202) -> ("QMH UI References.Refnum EXPERT"=w206:refnum<vi>)
        n87 = call "Gui_SetupExpert.vi"("error in (no error)"=w209, "QMH UI References.Refnum EXPERT"=w206) -> ("error out"=w204:errorcluster)  [unwired: 9 in]
        n88 = call "UI_Update_Status.vi"("error in (no error)"=w204, "UI Status"=QMH_UI_Command."Waiting for User", "QMH UI Cluster"=w202) -> ("error out"=w203:errorcluster)  [unwired: 6 in, 2 out]
      }
      frame "UI Change Scientist" {
        n89 = call "UI_Update_Status.vi"("error in (no error)"=w221, "UI Status"=w220, "QMH UI Cluster"=w217) -> ("error out"=w214:errorcluster, "Variant"=w212:variant, "QMH UI Cluster"=w210:T31)  [unwired: 6 in]
        n90 = call "QMH_UI_Control_EnQueue.vi"("error in (no error)"=w214, "Variant"=w212, "Command"=QMH_UI_Command."Update Report", "UI Queue"=w215) -> ("error out"=w213:errorcluster)  [unwired: 6 in, 1 out]
        n91 = call "Gui_SetupTimingTable.vi"("error in (no error)"=w213, "QMH UI Cluster"=w210) -> ("error out"=w222:errorcluster)  [unwired: 9 in]
        n92 = call "Gui_SetupTimingScript_Ions.vi"("error in (no error)"=w222, "QMH UI Cluster"=w210) -> ("error out"=w211:errorcluster)  [unwired: 9 in]
        n93 = call "UI_Update_Status.vi"("error in (no error)"=w211, "UI Status"=QMH_UI_Command."Waiting for User", "QMH UI Cluster"=w210) -> ("error out"=w219:errorcluster)  [unwired: 6 in, 2 out]
      }
      frame "UI Exit" {
        # "Generate the user event \"User Stop\" to stop the Loop of UI Events"
        n94 = call "QMH_ICR_Control_EnQueue.vi"("error in (no error)"=w227, "Command"=QMH_ICR_Command."Exit", "ICR Queue"=w224) -> ("error out"=w226:errorcluster)  [unwired: 7 in, 1 out]
        n95 = Release Queue(queue=w225, error in (no error)=w226) -> (error out=w233:errorcluster)  [unwired: 1 in, 2 out]
        n96 = Generate User Event(user event=w231, event data cluster=TRUE ("données d'événement")) -> (error out=w230:errorcluster)  [unwired: 2 in, 1 out]
        n97 = Merge Errors(w230, w233) -> (w229:errorcluster)
      }
      frame "Update Report" {
        w246 = T33 {"UI Status"=enum."Initialize", "ICR Status"=enum."Initialize", "QMH Status"=enum."Init"}  # QMH UI Report
        n98 = Variant To Data(error in=w242, type=w246, Variant=w247) -> (data=w239:T33, error out=w245:errorcluster)
        n99 = Bundle By Name(cluster=w237, "QMH UI Report"=w239) -> (w238:T31)
        n100 = Unbundle By Name(w239) -> ("UI Status"=w236:T34, "ICR Status"=w235:T35)  [unwired: 1 out]
        n101 = Unbundle By Name(w238) -> ("QMH UI References"=w240:T32)
        n102 = call "UI_Update_Controls.vi"("error in (no error)"=w245, "ICR Status"=w235, "UI Status"=w236, "QMH UI References"=w240) -> ("error out"=w241:errorcluster, "QMH UI References"=w244:T32)  [unwired: 6 in]
        n103 = Bundle By Name(cluster=w237, "QMH UI References"=w244) -> (w243:T31)
      }
      frame "Update ICR Status" {
        n104 = Variant To Data(error in=w260, type=QMH_ICR_Command."Initialize" ("Command"), Variant=w261) -> (data=w257:T35, error out=w253:errorcluster)
        n105 = Bundle By Name(cluster=w259, "QMH UI Report.ICR Status"=w257) -> (w250:T31)
        n106 = call "UI_Update_Status.vi"("error in (no error)"=w253, "UI Status"=QMH_UI_Command."Waiting for ICR", "QMH UI Cluster"=w250) -> ("error out"=w252:errorcluster, "Variant"=w249:variant, "QMH UI Cluster"=w251:T31)  [unwired: 6 in]
        n107 = call "QMH_UI_Control_EnQueue.vi"("error in (no error)"=w252, "Variant"=w249, "Command"=QMH_UI_Command."Update Report", "UI Queue"=w254) -> ("error out"=w255:errorcluster)  [unwired: 6 in, 1 out]
      }
      frame "Ready to Start" {
        n108 = call "UI_Update_Status.vi"("error in (no error)"=w265, "UI Status"=w266, "QMH UI Cluster"=w267) -> ("error out"=w269:errorcluster, "Variant"=w268:variant, "QMH UI Cluster"=w263:T31)  [unwired: 6 in]
        n109 = call "QMH_UI_Control_EnQueue.vi"("error in (no error)"=w269, "Variant"=w268, "Command"=QMH_UI_Command."Update Report", "UI Queue"=w264) -> ("error out"=w262:errorcluster)  [unwired: 6 in, 1 out]
      }
      frame "Waiting for ICR" {
        n110 = call "UI_Update_Status.vi"("error in (no error)"=w280, "UI Status"=w281, "QMH UI Cluster"=w282) -> ("error out"=w284:errorcluster, "Variant"=w283:variant, "QMH UI Cluster"=w271:T31)  [unwired: 6 in]
        n111 = To Variant(anything=w271) -> (Variant=w276:variant)
        n112 = call "QMH_UI_Control_EnQueue.vi"("error in (no error)"=w284, "Variant"=w283, "Command"=QMH_UI_Command."Update Report", "UI Queue"=w279) -> ("error out"=w275:errorcluster)  [unwired: 6 in, 1 out]
        n113 = call "QMH_ICR_Control_EnQueue.vi"("error in (no error)"=w275, "Variant"=w276, "Command"=QMH_ICR_Command."Sequence Setup", "ICR Queue"=w277) -> ("error out"=w273:errorcluster)  [unwired: 6 in, 1 out]
        n114 = call "UI_Update_Status.vi"("error in (no error)"=w273, "UI Status"=QMH_UI_Command."Waiting for ICR", "QMH UI Cluster"=w271) -> ("error out"=w272:errorcluster)  [unwired: 6 in, 2 out]
      }
      frame Default {
        (unwired) errorcluster {"status"=FALSE, "code"=0, "source"=""} ("sortie d'erreur")
        # "La condition 'Par défaut' ne s'exécute que s'il y a un message qui n'est défini dans aucune des autres conditions.  Renvoyer une erreur."
        n115 = One Button Dialog(message="Invalid Message") -> ()  [unwired: 1 in, 1 out]
      }
    }
  }
  n116 = while "Producer Loop for UI events" {
    tunnel: w11 -> [w294]
    tunnel: [w288] -> w21
    shift-right: [w290] -> w20
    shift-left: w24 -> [w291]
    stop <- w295 stop-if-true
    # "Error : send a message Exit to\nthe top of the queue"
    n117 = event shown="[0] \"Load\": Valeur changée" {
      selector: w291 -> [_ _ _ _ _ _ _ _ _ _ _ _]
      dyn-events: [_ _ _ _ _ _ _ _ _ _ _ _] -> w290
      timeout: _ -> [_ _ _ _ _ _ _ _ _ _ _ _]
      tunnel: w294 -> [w298 w301 w304 w308 w312 w316 w322 w326 w331 w335 w343 w345]
      tunnel: [w296 w302 w305 w309 w313 w317 w320 w324 w330 w334 w342 _] -> w293
      tunnel: [w297 w303 w306 w310 w314 w318 w321 w325 w329 w333 w343 w345] -> w292
      tunnel: [_ _ _ _ _ _ _ _ _ _ _ TRUE ("User Stop")] -> w289
      event "Load": Value Change {
        n118 = event-data() -> ()  [unwired: 2 out]
        n119 = call "QMH_UI_Control_EnQueue.vi"("Command"=QMH_UI_Command."UI Load", "UI Queue"=w298) -> ("error out"=w296:errorcluster, "UI Queue"=w297:refnum<queue>)  [unwired: 8 in]
      }
      event "Change Experiment": Value Change {
        n120 = event-data() -> ()  [unwired: 2 out]
        n121 = call "QMH_UI_Control_EnQueue.vi"("Command"=QMH_UI_Command."UI Change Experiment", "UI Queue"=w301) -> ("error out"=w302:errorcluster, "UI Queue"=w303:refnum<queue>)  [unwired: 8 in]
      }
      event "Change Voltages": Value Change {
        n122 = event-data() -> ()  [unwired: 2 out]
        n123 = call "QMH_UI_Control_EnQueue.vi"("Command"=QMH_UI_Command."UI Change Voltages", "UI Queue"=w304) -> ("error out"=w305:errorcluster, "UI Queue"=w306:refnum<queue>)  [unwired: 8 in]
      }
      event "Change Sequence": Value Change {
        n124 = event-data() -> ()  [unwired: 2 out]
        n125 = call "QMH_UI_Control_EnQueue.vi"("Command"=QMH_UI_Command."UI Change Sequence", "UI Queue"=w308) -> ("error out"=w309:errorcluster, "UI Queue"=w310:refnum<queue>)  [unwired: 8 in]
      }
      event "Change Expert": Value Change {
        n126 = event-data() -> ()  [unwired: 2 out]
        n127 = call "QMH_UI_Control_EnQueue.vi"("Command"=QMH_UI_Command."UI Change Expert", "UI Queue"=w312) -> ("error out"=w313:errorcluster, "UI Queue"=w314:refnum<queue>)  [unwired: 8 in]
      }
      event "Change Scientist": Value Change {
        n128 = event-data() -> ()  [unwired: 2 out]
        n129 = call "QMH_UI_Control_EnQueue.vi"("Command"=QMH_UI_Command."UI Change Scientist", "UI Queue"=w316) -> ("error out"=w317:errorcluster, "UI Queue"=w318:refnum<queue>)  [unwired: 8 in]
      }
      event "Save As": Value Change {
        n130 = event-data() -> ()  [unwired: 2 out]
        n131 = call "QMH_UI_Control_EnQueue.vi"("Command"=QMH_UI_Command."UI Save As", "UI Queue"=w322) -> ("error out"=w320:errorcluster, "UI Queue"=w321:refnum<queue>)  [unwired: 8 in]
      }
      event "Start": Value Change {
        n132 = event-data() -> ()  [unwired: 2 out]
        n133 = call "QMH_UI_Control_EnQueue.vi"("Command"=QMH_UI_Command."UI Start", "UI Queue"=w326) -> ("error out"=w324:errorcluster, "UI Queue"=w325:refnum<queue>)  [unwired: 8 in]
      }
      event "Exit": Value Change {
        n134 = event-data() -> ()  [unwired: 2 out]
        n135 = call "QMH_UI_Control_EnQueue.vi"("Command"=QMH_UI_Command."UI Exit", "UI Queue"=w331) -> ("error out"=w330:errorcluster, "UI Queue"=w329:refnum<queue>)  [unwired: 8 in]
      }
      event Menu Selection (User) {
        n136 = event-data() -> ("ItemTag"=w332:string)  [unwired: 1 out]
        n137 = case shown="\"Exit\"" w332 {
          tunnel: w335 -> [w339 w340]
          tunnel: [w337 w341] -> w334
          tunnel: [w338 w340] -> w333
          frame "Exit" {
            n138 = call "QMH_UI_Control_EnQueue.vi"("Command"=QMH_UI_Command."UI Exit", "UI Queue"=w339) -> ("error out"=w337:errorcluster, "UI Queue"=w338:refnum<queue>)  [unwired: 8 in]
          }
          frame "About", Default {
            n139 = call "Gui_About.vi"() -> ("error out"=w341:errorcluster)  [unwired: 11 in]
          }
        }
      }
      event "Excit Test": Value Change {
        n140 = event-data() -> ()  [unwired: 2 out]
        n141 = call "Hard_AWG_5421_Standard_Function.vi"() -> ("error out"=w342:errorcluster)  [unwired: 11 in]
      }
      event User Event {
        n142 = event-data() -> ()  [unwired: 3 out]
      }
    }
    n143 = case shown="Pas d'erreur" w293 {
      selector: w293 -> [w346 _]
      tunnel: [w347 TRUE] -> w295
      tunnel: w292 -> [_ w351]
      tunnel: w289 -> [w347 _]
      tunnel: [w346 w348] -> w288
      frame No Error {
      }
      frame Error {
        n144 = call "QMH_UI_Control_EnQueue.vi"("Last ?"=FALSE, "Command"=QMH_UI_Command."UI Exit", "UI Queue"=w351) -> ("error out"=w348:errorcluster)  [unwired: 7 in, 1 out]
      }
    }
  }
  n145 = Unregister For Events(event registration refnum=w20, error in=w21) -> (error out=w17:errorcluster)
  n146 = Destroy User Event(user event=w18, error in=w17) -> (error out=w16:errorcluster)
  n147 = Merge Errors(w16, w19, w9) -> (w12:errorcluster)
  n148 = property on="Property Node" class="App"(error in=w12) -> (error out=w15:errorcluster, "App.Kind"=w14:T40)  [unwired: 1 in, 1 out]
  n149 = call <vilib>:"Simple Error Handler.vi"("error in (no error)"=w15) -> ("error out"=w13:errorcluster)  [unwired: 4 in, 4 out]
  n150 = case shown="\"Run Time System\"" w14 {
    tunnel: w13 -> [_ _]
    frame Default {
    }
    frame "Run Time System" {
      n151 = Quit LabVIEW() -> ()  [unwired: 1 in]
    }
  }
